vi "Command.vi"(8 "error in (no error)":errorcluster, 9 "data in":u8[](array[numeric]) format="%x", 10 "function code":u8=1 format="%x", 11 "MODBUS in":refnum<class "PL Modbus Client.lvclass">) -> (0 "error out":errorcluster, 2 "data out":u8[](array[numeric]) format="%x", 3 "MODBUS out":refnum<class "PL Modbus Client.lvclass">)   [LabVIEW 2015, in "PL Modbus Client.lvclass"]
doc: "Sends Modbus request with specified <B>function code</B> and <B>data in</B> and returns response data as <B>data out</B>. For not implemented function codes used via Modbus RTU <B>read RTU data callback</B> should be provided (default Read RTU Data.vi can be used as a template)."
uses:
  PL Modbus Client.lvclass
  PL Modbus Client.lvclass/PL Modbus Client.ctl
panel:
  out "exception":bool
  out "read buffer":string
  out "VISA locked":bool
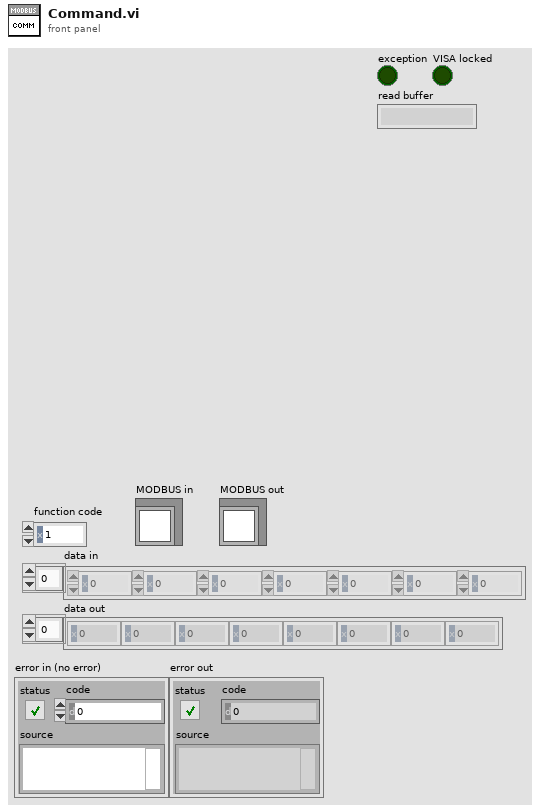
[diagram p1: front panel]
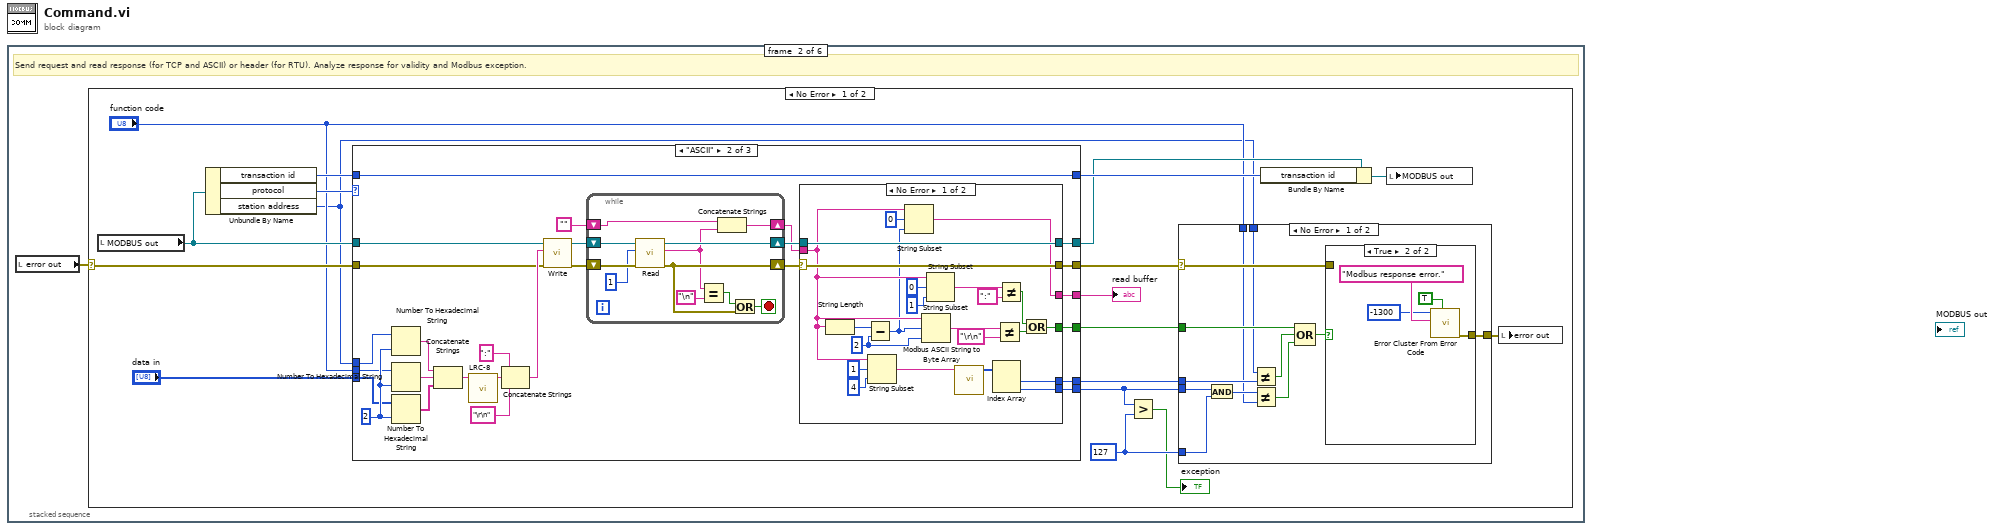
[diagram p0: block diagram]
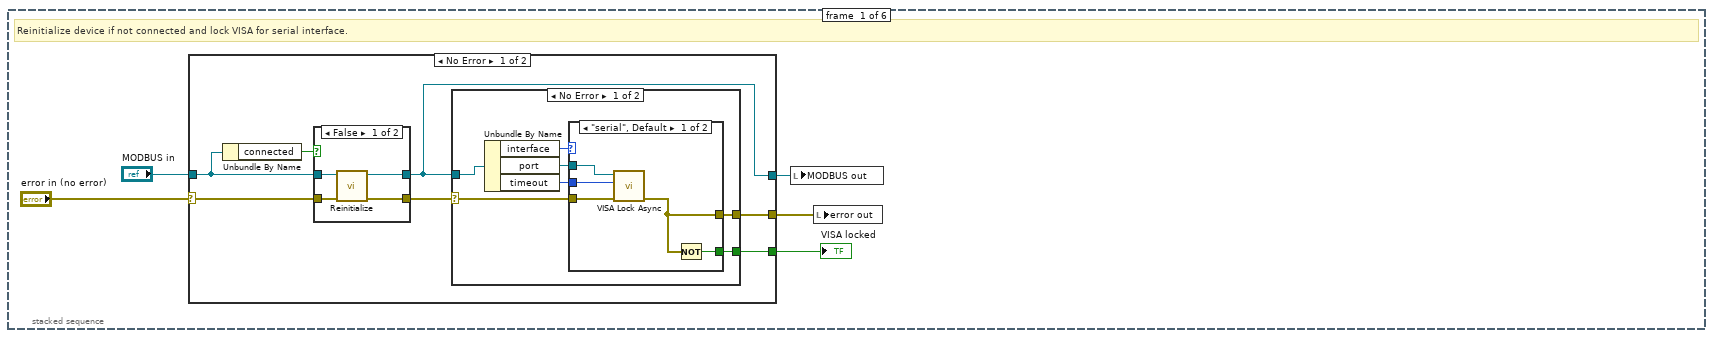
[diagram p2: hidden frame]
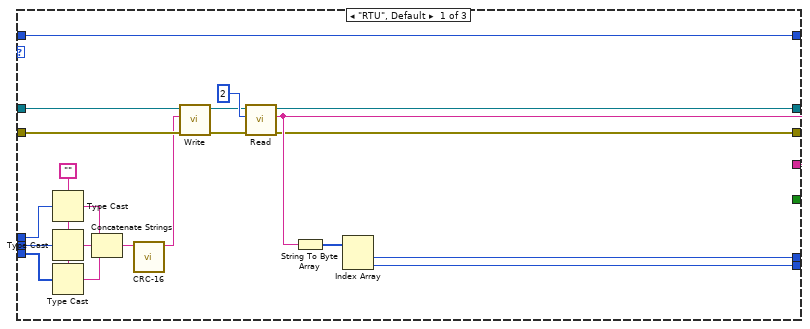
[diagram p9: hidden frame]
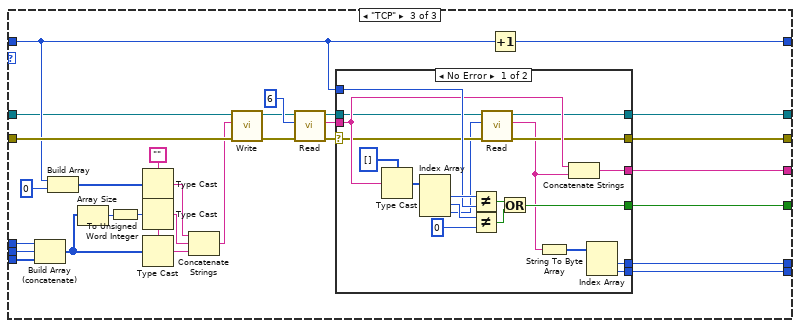
[diagram p11: hidden frame]
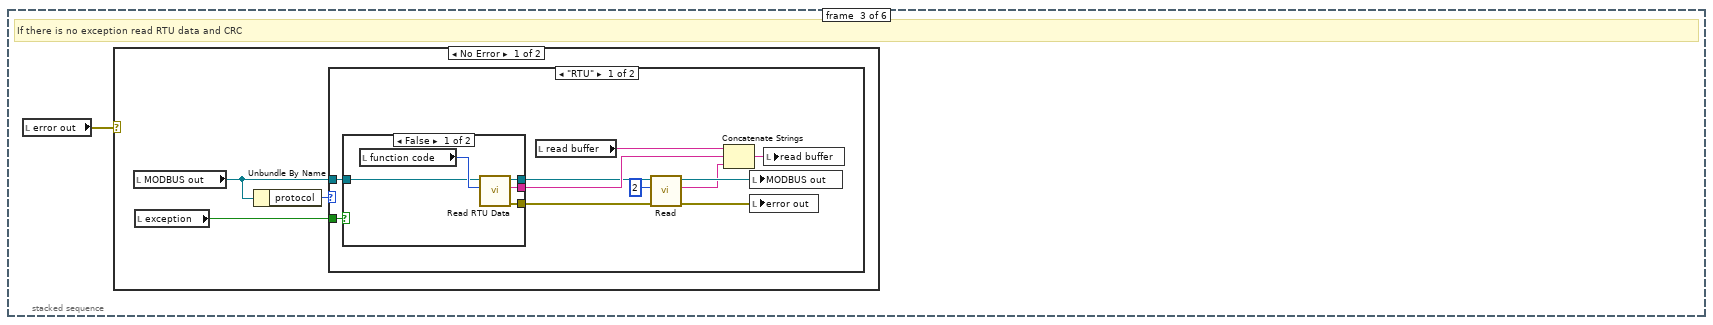
[diagram p14: hidden frame]
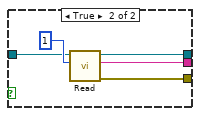
[diagram p15: hidden frame]
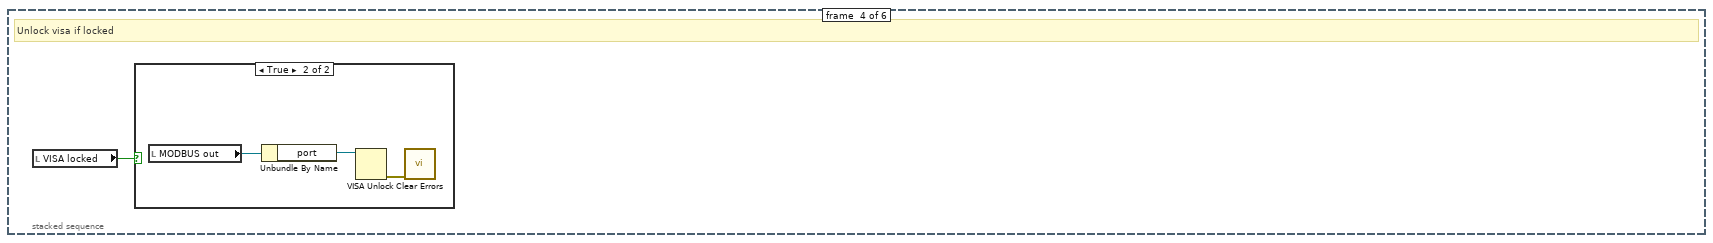
[diagram p18: hidden frame]
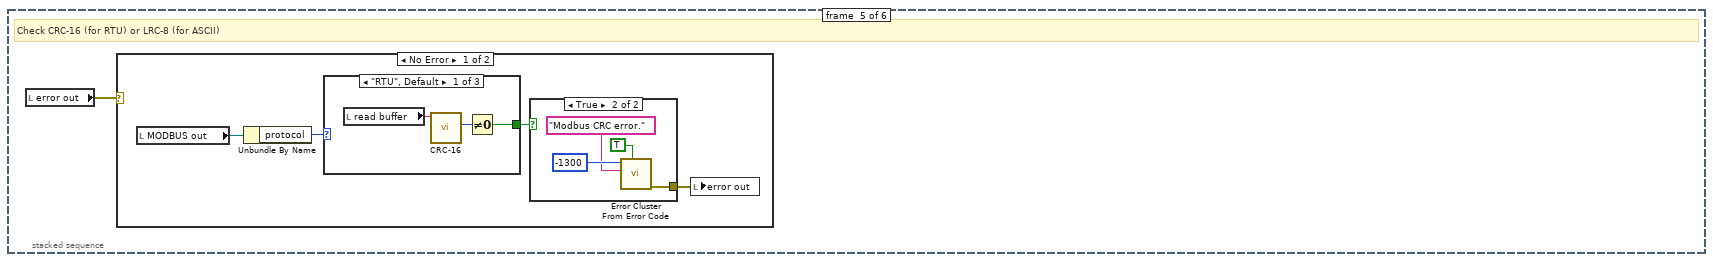
[diagram p20: hidden frame]
diagram:
  n1 = stacked-sequence {
    frame #0 {
      # "Reinitialize device if not connected and lock VISA for serial interface."
      n2 = case shown="No Error" "error in (no error)" {
        selector: "error in (no error)" -> [w7 w33]
        tunnel: [w12 _] -> w5
        tunnel: [w11 w33] -> w4
        tunnel: "MODBUS in" -> [w9 w34]
        tunnel: [w6 w34] -> w2
        frame No Error {
          n3 = Unbundle By Name(w9) -> ("connected"=w10:bool)
          n4 = case shown="False" w10 {
            tunnel: w9 -> [w16 w18]
            tunnel: [w15 w18] -> w6
            tunnel: w7 -> [w13 w17]
            tunnel: [w14 w17] -> w8
            frame False {
              n5 = call "Reinitialize.vi"("error in (no error)"=w13, "MODBUS in"=w16) -> ("error out"=w14:errorcluster, "MODBUS out"=w15:refnum<class "PL Modbus Client.lvclass">)  [unwired: 8 in]
            }
            frame True {
            }
          }
          n6 = case shown="No Error" w8 {
            selector: w8 -> [w19 w32]
            tunnel: w6 -> [w24 _]
            tunnel: [w21 _] -> w12
            tunnel: [w20 w32] -> w11
            frame No Error {
              n7 = Unbundle By Name(w24) -> ("interface"=w25:enum16{"serial", "network"}, "port"=w23:refnum<visa-resource-name>, "timeout"=w22:u32)
              n8 = case shown="\"serial\", Default" w25 {
                tunnel: w23 -> [w30 _]
                tunnel: w22 -> [w29 _]
                tunnel: [w28 _] -> w21
                tunnel: [w27 w31] -> w20
                tunnel: w19 -> [w26 w31]
                frame "serial", Default {
                  n9 = call <vilib>:"VISA Lock Async.vi"("error in (no error)"=w26, "timeout (0)"=w29, "VISA resource name"=w30) -> ("error out"=w27:errorcluster)  [unwired: 6 in, 2 out]
                  n10 = Not(x=w27) -> (.not. x?=w28:bool)
                }
                frame "network" {
                }
              }
            }
            frame Error {
            }
          }
        }
        frame Error {
        }
      }
      "VISA locked" <- w5
      n11 = local write "MODBUS out"(w2) -> ()
      n12 = local write "error out"(w4) -> ()
    }
    frame #1 {
      # "Send request and read response (for TCP and ASCII) or header (for RTU). Analyze response for validity and Modbus exception."
      n13 = local read "error out"() -> (w35:errorcluster)
      n14 = case shown="No Error" w35 {
        selector: w35 -> [w41 _]
        frame No Error {
          w47 = u8 127
          n15 = local read "MODBUS out"() -> (w42:refnum<class "PL Modbus Client.lvclass">)
          n16 = Unbundle By Name(w42) -> ("transaction id"=w52:u16, "protocol"=w40:enum16{"RTU", "ASCII", "TCP"}, "station address"=w36:u8)
          n17 = case shown="\"ASCII\"" w40 {
            tunnel: w41 -> [w76 w94 w162]
            tunnel: [w73 w118 w183] -> w51
            tunnel: [w88 w109 w182] -> w39
            tunnel: [w92 w119 w184] -> w53
            tunnel: w52 -> [w92 w119 w157]
            tunnel: [w91 w115 w181] -> w49
            tunnel: [w90 w114 w180] -> w48
            tunnel: [_ w117 w179] -> w50
            tunnel: [w87 w116 w178] -> w43
            tunnel: w42 -> [w74 w93 w156]
            tunnel: "data in" -> [w78 w96 w164]
            tunnel: "function code" -> [w80 w98 w161]
            tunnel: w36 -> [w79 w97 w160]
            frame "RTU", Default {
              w81 = ""
              n18 = Type Cast(type=w81, x=w79) -> (*(type *) &x=w82:string)
              n19 = Type Cast(type=w81, x=w80) -> (*(type *) &x=w83:string)
              n20 = Type Cast(type=w81, x=w78) -> (*(type *) &x=w84:string)
              n21 = Concatenate Strings(w82, w83, w84) -> (w85:string)
              n22 = call "CRC-16.vi"("string"=w85) -> ("string with CRC-16"=w75:string)  [unwired: 9 in, 1 out]
              n23 = call "Write.vi"("error in (no error)"=w76, "write buffer"=w75, "MODBUS in"=w74) -> ("error out"=w72:errorcluster, "MODBUS out"=w77:refnum<class "PL Modbus Client.lvclass">)  [unwired: 7 in]
              n24 = call "Read.vi"("error in (no error)"=w72, "byte count"=u32 2, "MODBUS in"=w77) -> ("error out"=w73:errorcluster, "read buffer"=w87:string, "MODBUS out"=w88:refnum<class "PL Modbus Client.lvclass">)  [unwired: 6 in]
              n25 = String To Byte Array(string=w87) -> (unsigned byte array=w89:u8[])
              n26 = Index Array(array=w89) -> (element #1=w91:u8, element #2=w90:u8)  [unwired: 2 in]
            }
            frame "ASCII" {
              w102 = 2
              n27 = Number To Hexadecimal String(1:w102, 2:w97) -> (0:w106:string)
              n28 = Number To Hexadecimal String(1:w102, 2:w98) -> (0:w105:string)
              n29 = Number To Hexadecimal String(1:w102, 2:w96) -> (0:w99:string[])
              n30 = Concatenate Strings(w106, w105, w99) -> (w101:string)
              n31 = call "LRC-8.vi"("string"=w101) -> ("string with LRC-8"=w100:string)  [unwired: 9 in, 1 out]
              n32 = Concatenate Strings(":", w100, "\r\n") -> (w95:string)
              n33 = call "Write.vi"("error in (no error)"=w94, "write buffer"=w95, "MODBUS in"=w93) -> ("error out"=w107:errorcluster, "MODBUS out"=w108:refnum<class "PL Modbus Client.lvclass">)  [unwired: 7 in]
              n34 = while {
                shift-right: [w126] -> w113
                shift-left: w107 -> [w128]
                shift-right: [w129] -> w112
                shift-left: w108 -> [w130]
                shift-right: [w121] -> w110
                shift-left: "" -> [w120]
                stop <- w125 stop-if-true
                n35 = call "Read.vi"("error in (no error)"=w128, "byte count"=u32 1, "MODBUS in"=w130) -> ("error out"=w126:errorcluster, "read buffer"=w122:string, "MODBUS out"=w129:refnum<class "PL Modbus Client.lvclass">)  [unwired: 6 in]
                n36 = Equal?(x=w122, y="\n") -> (x = y?=w123:bool)
                n37 = Concatenate Strings(w120, w122) -> (w121:string)
                n38 = Or(x=w123, y=w126) -> (x .or. y?=w125:bool)
              }
              n39 = case shown="No Error" w113 {
                selector: w113 -> [w148 w155]
                tunnel: w112 -> [w152 w154]
                tunnel: [w148 w155] -> w118
                tunnel: [w152 w154] -> w109
                tunnel: w110 -> [w134 _]
                tunnel: [w138 _] -> w117
                tunnel: [w151 _] -> w115
                tunnel: [w150 _] -> w114
                tunnel: [w131 _] -> w116
                frame No Error {
                  w139 = 2 ("y")
                  n40 = String Length(string=w134) -> (length=w140:i32)
                  n41 = Subtract(x=w140, y=w139) -> (x-y=w132:i32)
                  n42 = String Subset(string=w134, offset (0)=1, length (rest)=4 ("length (rest)")) -> (substring=w141:string)
                  n43 = String Subset(string=w134, offset (0)=0, length (rest)=w132) -> (substring=w131:string)
                  n44 = String Subset(string=w134, offset (0)=w132, length (rest)=w139) -> (substring=w137:string)
                  n45 = String Subset(string=w134, offset (0)=0, length (rest)=1 ("length (rest)")) -> (substring=w146:string)
                  n46 = call "Modbus ASCII String to Byte Array.vi"("string"=w141) -> ("byte array"=w149:u8[])  [unwired: 10 in]
                  n47 = Index Array(array=w149) -> (element #1=w151:u8, element #2=w150:u8)  [unwired: 2 in]
                  n48 = Not Equal?(x=w137, y="\r\n") -> (x != y?=w136:bool)
                  n49 = Not Equal?(x=w146, y=":") -> (x != y?=w147:bool)
                  n50 = Or(x=w147, y=w136) -> (x .or. y?=w138:bool)
                }
                frame Error {
                }
              }
            }
            frame "TCP" {
              w168 = ""
              n51 = Build Array (concatenate)(w160, w161, w164) -> (w171:u8[])
              n52 = Build Array(w157, u16 0 ("element")) -> (w169:u16[])
              n53 = Array Size(array=w171) -> (size(s)=w172:i32)
              n54 = To Unsigned Word Integer(number=w172) -> (unsigned 16bit integer=w173:u16)
              n55 = Type Cast(type=w168, x=w169) -> (*(type *) &x=w170:string)
              n56 = Type Cast(type=w168, x=w173) -> (*(type *) &x=w165:string)
              n57 = Type Cast(type=w168, x=w171) -> (*(type *) &x=w166:string)
              n58 = Concatenate Strings(w170, w165, w166) -> (w158:string)
              n59 = call "Write.vi"("error in (no error)"=w162, "write buffer"=w158, "MODBUS in"=w156) -> ("error out"=w159:errorcluster, "MODBUS out"=w163:refnum<class "PL Modbus Client.lvclass">)  [unwired: 7 in]
              n60 = call "Read.vi"("error in (no error)"=w159, "byte count"=u32 6 ("bytes to read"), "MODBUS in"=w163) -> ("error out"=w177:errorcluster, "read buffer"=w174:string, "MODBUS out"=w175:refnum<class "PL Modbus Client.lvclass">)  [unwired: 6 in]
              n61 = case shown="No Error" w177 {
                selector: w177 -> [w189 w206]
                tunnel: [w188 w206] -> w183
                tunnel: w174 -> [w191 _]
                tunnel: w175 -> [w190 w205]
                tunnel: [w187 w205] -> w182
                tunnel: w157 -> [w198 _]
                tunnel: [w195 _] -> w181
                tunnel: [w194 _] -> w180
                tunnel: [w193 _] -> w179
                tunnel: [w192 _] -> w178
                frame No Error {
                  n62 = Type Cast(type=u16[] [], x=w191) -> (*(type *) &x=w203:u16[])
                  n63 = Index Array(array=w203) -> (element #1=w202:u16, element #2=w201:u16, element #3=w186:u16)  [unwired: 3 in]
                  n64 = Not Equal?(x=w202, y=w198) -> (x != y?=w197:bool)
                  n65 = Not Equal?(x=w201, y=u16 0) -> (x != y?=w196:bool)
                  n66 = call "Read.vi"("error in (no error)"=w189, "byte count"=w186, "MODBUS in"=w190) -> ("error out"=w188:errorcluster, "read buffer"=w185:string, "MODBUS out"=w187:refnum<class "PL Modbus Client.lvclass">)  [unwired: 6 in]
                  n67 = Or(x=w197, y=w196) -> (x .or. y?=w193:bool)
                  n68 = String To Byte Array(string=w185) -> (unsigned byte array=w199:u8[])
                  n69 = Concatenate Strings(w191, w185) -> (w192:string)
                  n70 = Index Array(array=w199) -> (element #1=w195:u8, element #2=w194:u8)  [unwired: 2 in]
                }
                frame Error {
                }
              }
              n71 = Increment(x=w157) -> (x+1=w184:u16)
            }
          }
          "read buffer" <- w43
          n72 = Greater?(x=w48, y=w47) -> (0:→"exception":bool)
          n73 = case shown="No Error" w51 {
            selector: w51 -> [w61 w71]
            tunnel: [w65 w71] -> w44
            tunnel: w50 -> [w60 _]
            tunnel: w49 -> [w57 _]
            tunnel: w48 -> [w56 _]
            tunnel: w36 -> [w55 _]
            tunnel: w47 -> [w63 _]
            tunnel: "function code" -> [w54 _]
            frame No Error {
              n74 = And(x=w56, y=w63) -> (x .and. y?=w62:u8)
              n75 = Not Equal?(x=w55, y=w57) -> (x != y?=w59:bool)
              n76 = Not Equal?(x=w62, y=w54) -> (x != y?=w58:bool)
              n77 = Compound Arithmetic op=OR(w60, w59, w58) -> (w64:bool)
              n78 = case shown="True" w64 {
                tunnel: [w66 w68] -> w65
                tunnel: w61 -> [w66 _]
                frame False {
                }
                frame True {
                  n79 = call <vilib>:"Error Cluster From Error Code.vi"("show call chain? (False)"=TRUE, "error message (\"\")"="Modbus response error." ("format string"), "error code (0)"=-1300) -> ("error out"=w68:errorcluster)  [unwired: 6 in]
                }
              }
            }
            frame Error {
            }
          }
          n80 = Bundle By Name(cluster=w39, "transaction id"=w53) -> (w45:refnum<class "PL Modbus Client.lvclass">)
          n81 = local write "MODBUS out"(w45) -> ()
          n82 = local write "error out"(w44) -> ()
        }
        frame Error {
        }
      }
    }
    frame #2 {
      # "If there is no exception read RTU data and CRC"
      n83 = local read "error out"() -> (w207:errorcluster)
      n84 = case shown="No Error" w207 {
        frame No Error {
          n85 = local read "MODBUS out"() -> (w210:refnum<class "PL Modbus Client.lvclass">)
          n86 = local read "exception"() -> (w209:bool)
          n87 = Unbundle By Name(w210) -> ("protocol"=w208:enum16{"RTU", "ASCII", "TCP"})
          n88 = case shown="\"RTU\"" w208 {
            tunnel: w210 -> [w221 _]
            tunnel: w209 -> [w220 _]
            frame "RTU" {
              n89 = case shown="False" w220 {
                tunnel: w221 -> [w225 w230]
                tunnel: [w224 w229] -> w216
                tunnel: [w223 w228] -> w215
                tunnel: [w222 w227] -> w217
                frame False {
                  n90 = local read "function code"() -> (w226:u8)
                  n91 = call-dynamic "Read RTU Data.vi"("function code"=w226, "MODBUS in"=w225) -> ("error out"=w223:errorcluster, "data"=w222:string, "MODBUS out"=w224:refnum<class "PL Modbus Client.lvclass">)  [unwired: 7 in]
                }
                frame True {
                  n92 = call "Read.vi"("byte count"=u32 1 ("data byte count"), "MODBUS in"=w230) -> ("error out"=w228:errorcluster, "read buffer"=w227:string, "MODBUS out"=w229:refnum<class "PL Modbus Client.lvclass">)  [unwired: 7 in]
                }
              }
              n93 = local read "read buffer"() -> (w219:string)
              n94 = call "Read.vi"("error in (no error)"=w215, "byte count"=u32 2 ("data byte count"), "MODBUS in"=w216) -> ("error out"=w212:errorcluster, "read buffer"=w211:string, "MODBUS out"=w213:refnum<class "PL Modbus Client.lvclass">)  [unwired: 6 in]
              n95 = Concatenate Strings(w219, w217, w211) -> (w218:string)
              n96 = local write "MODBUS out"(w213) -> ()
              n97 = local write "error out"(w212) -> ()
              n98 = local write "read buffer"(w218) -> ()
            }
            frame "ASCII", Default {
            }
          }
        }
        frame Error {
        }
      }
    }
    frame #3 {
      # "Unlock visa if locked"
      n99 = local read "VISA locked"() -> (w232:bool)
      n100 = case shown="True" w232 {
        frame False {
        }
        frame True {
          n101 = local read "MODBUS out"() -> (w235:refnum<class "PL Modbus Client.lvclass">)
          n102 = Unbundle By Name(w235) -> ("port"=w233:refnum<visa-resource-name>)
          n103 = VISA Unlock(11:w233) -> (0:w234:errorcluster)  [unwired: 1 in, 1 out]
          n104 = call <vilib>:"Clear Errors.vi"("error in (no error)"=w234) -> ()  [unwired: 5 in, 2 out]
        }
      }
    }
    frame #4 {
      # "Check CRC-16 (for RTU) or LRC-8 (for ASCII)"
      n105 = local read "error out"() -> (w236:errorcluster)
      n106 = case shown="No Error" w236 {
        frame No Error {
          n107 = local read "MODBUS out"() -> (w240:refnum<class "PL Modbus Client.lvclass">)
          n108 = Unbundle By Name(w240) -> ("protocol"=w239:enum16{"RTU", "ASCII", "TCP"})
          n109 = case shown="\"RTU\", Default" w239 {
            tunnel: [w243 w244 _] -> w237
            frame "RTU", Default {
              n110 = local read "read buffer"() -> (w242:string)
              n111 = call "CRC-16.vi"("string"=w242) -> ("CRC-16"=w241:u16)  [unwired: 9 in, 1 out]
              n112 = Not Equal To 0?(x=w241) -> (x != 0?=w243:bool)
            }
            frame "ASCII" {
              n113 = local read "read buffer"() -> (w245:string)
              n114 = call "LRC-8.vi"("string"=w245) -> ("LRC-8"=w246:u8)  [unwired: 9 in, 1 out]
              n115 = Not Equal To 0?(x=w246) -> (x != 0?=w244:bool)
            }
            frame "TCP" {
            }
          }
          n116 = case shown="True" w237 {
            tunnel: [_ w248] -> w238
            frame False {
            }
            frame True {
              n117 = call <vilib>:"Error Cluster From Error Code.vi"("show call chain? (False)"=TRUE, "error message (\"\")"="Modbus CRC error." ("format string"), "error code (0)"=-1300) -> ("error out"=w248:errorcluster)  [unwired: 6 in]
            }
          }
          n118 = local write "error out"(w238) -> ()
        }
        frame Error {
        }
      }
    }
    frame #5 {
      # "Convert data to U8 / Create Modbus exception error cluster / Set client state as \"not connected\""
      n119 = local read "MODBUS out"() -> (w251:refnum<class "PL Modbus Client.lvclass">)
      n120 = local read "error out"() -> (w252:errorcluster)
      n121 = case shown="No Error" w252 {
        selector: w252 -> [_ w299]
        tunnel: w251 -> [_ w298]
        frame No Error {
          n122 = local read "MODBUS out"() -> (w258:refnum<class "PL Modbus Client.lvclass">)
          n123 = local read "read buffer"() -> (w257:string)
          n124 = Unbundle By Name(w258) -> ("protocol"=w253:enum16{"RTU", "ASCII", "TCP"})
          n125 = case shown="\"TCP\"" w253 {
            tunnel: w257 -> [w281 w288 w290]
            tunnel: [w280 w287 w289] -> w255
            frame "RTU", Default {
              n126 = String To Byte Array(string=w281) -> (unsigned byte array=w278:u8[])
              n127 = Array Size(array=w278) -> (size(s)=w277:i32)
              n128 = Subtract(x=w277, y=4) -> (x-y=w276:i32)
              n129 = Array Subset(array=w278, index=2, length=w276) -> (w280:u8[])
            }
            frame "ASCII" {
              n130 = String Length(string=w288) -> (length=w286:i32)
              n131 = Subtract(x=w286, y=7) -> (x-y=w284:i32)
              n132 = String Subset(string=w288, offset (0)=5, length (rest)=w284) -> (substring=w282:string)
              n133 = call "Modbus ASCII String to Byte Array.vi"("string"=w282) -> ("byte array"=w287:u8[])  [unwired: 10 in]
            }
            frame "TCP" {
              n134 = String To Byte Array(string=w290) -> (unsigned byte array=w294:u8[])
              n135 = Array Size(array=w294) -> (size(s)=w293:i32)
              n136 = Subtract(x=w293, y=8) -> (x-y=w292:i32)
              n137 = Array Subset(array=w294, index=8, length=w292) -> (w289:u8[])
            }
          }
          n138 = local read "exception"() -> (w256:bool)
          n139 = case shown="True" w256 {
            tunnel: w255 -> [w259 w274]
            tunnel: [w259 _] -> w254
            frame False {
            }
            frame True {
              w269 = ""
              n140 = Index Array(array=w274) -> (element=w261:u8)  [unwired: 1 in]
              n141 = Index Array(array=string[] ["", "ILLEGAL FUNCTION", "ILLEGAL DATA ADDRESS", "ILLEGAL DATA VALUE", "SERVER DEVICE FAILURE", "ACKNOWLEDGE", "SERVER DEVICE BUSY", "", "MEMORY PARITY ERROR", "", "GATEWAY PATH UNAVAILABLE", "GATEWAY TARGET DEVICE FAILED TO RESPOND"], index=w261) -> (element=w266:string)
              n142 = Not Equal?(x=w266, y=w269) -> (x != y?=w270:bool)
              n143 = Concatenate Strings(" (" ("string"), w266, ")" ("string")) -> (w265:string)
              n144 = Select(t=w265, s=w270, f=w269) -> (s? t:f=w263:string)
              n145 = Format Into String(format string="Modbus exception code 0x%02x%s.", w261, w263) -> (resulting string=w271:string)  [unwired: 2 in, 1 out]
              n146 = call <vilib>:"Error Cluster From Error Code.vi"("show call chain? (False)"=TRUE, "error message (\"\")"=w271, "error code (0)"=-1300) -> ("error out"=w260:errorcluster)  [unwired: 6 in]
              n147 = local write "error out"(w260) -> ()
            }
          }
          "data out" <- w254
        }
        frame Error {
          n148 = Unbundle By Name(w299) -> ("code"=w301:i32)
          n149 = Not Equal?(x=w301, y=-1300 ("error code (0)")) -> (x != y?=w300:bool)
          n150 = And(x=w299, y=w300) -> (x .and. y?=w297:bool)
          n151 = case shown="True" w297 {
            tunnel: w298 -> [w303 w306]
            tunnel: [w303 w304] -> w296
            frame False {
            }
            frame True {
              n152 = Bundle By Name(cluster=w306, "connected"=FALSE) -> (w304:refnum<class "PL Modbus Client.lvclass">)
            }
          }
          n153 = local write "MODBUS out"(w296) -> ()
        }
      }
    }
  }
